vi "build.vi"(8 "error in (no error)":errorcluster, 11 "PackedLibrary in":refnum<class "PackedLibrary.lvclass">) -> (0 "error out":errorcluster, 2 "GeneratedFiles":path[](array[path]), 3 "PackedLibrary out":refnum<class "PackedLibrary.lvclass">)   [LabVIEW 2024, in "PackedLibrary.lvclass"]
uses:
  PackedLibrary.lvclass
  PackedLibrary.lvclass/PackedLibrary.ctl
  <vilib>/AppBuilder/AB_API/PPL/NI_AB_API_PPL.lvclass
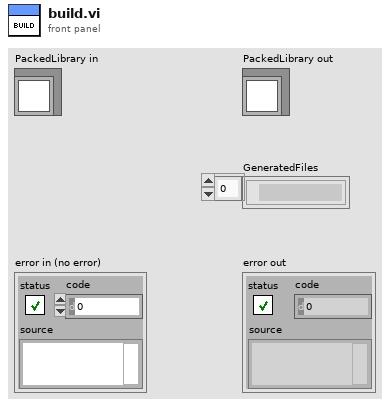
[diagram p1: front panel]
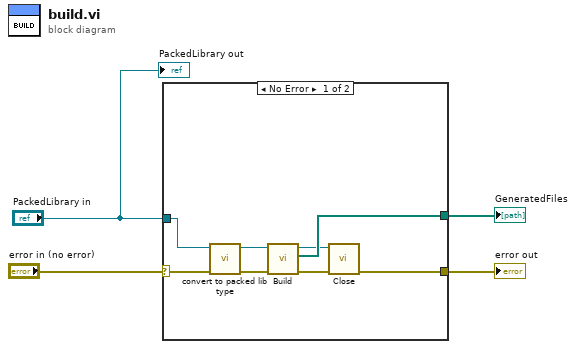
[diagram p0: block diagram]
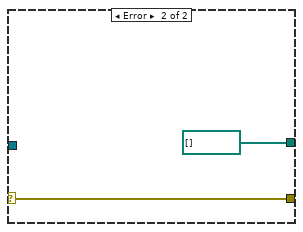
[diagram p2: hidden frame]
diagram:
  n1 = case shown="No Error" "error in (no error)" {
    selector: "error in (no error)" -> [w5 w14]
    tunnel: [w12 w14] -> w2
    tunnel: [w11 path[] [] ("GeneratedFiles")] -> w3
    tunnel: "PackedLibrary in" -> [w6 _]
    frame No Error {
      n2 = call "convert to packed lib type.vi"("error in (no error)"=w5, "PackedLibrary in"=w6) -> ("error out"=w8:errorcluster, "NI_AB_API_PPL out"=w7:refnum<class "NI_AB_API_PPL.lvclass">)  [unwired: 8 in]
      n3 = call-dynamic "Build.vi"("error in (no error)"=w8, "PPL in"=w7) -> ("error out"=w9:errorcluster, "GeneratedFiles"=w11:path[], "PPL out"=w10:refnum<class "NI_AB_API_PPL.lvclass">)  [unwired: 6 in, 1 out]
      n4 = call-dynamic "Close.vi"("error in (no error)"=w9, "DLL in"=w10) -> ("error out"=w12:errorcluster)  [unwired: 9 in]
    }
    frame Error {
    }
  }
  "error out" <- w2
  "GeneratedFiles" <- w3
  "PackedLibrary out" <- "PackedLibrary in"
